vi "GetFunctionOptions.vi"(9 "Function in":refnum<class "Function.lvclass">) -> (3 "Function out":refnum<class "Function.lvclass">, 4 "options":string)   [LabVIEW 2014, in "Raspberry Pi Compatible Compiler for LabVIEW.lvlib" / "Function.lvclass"]
uses:
  Function.lvclass
  Python/Parsing/Python Functions.lvlib
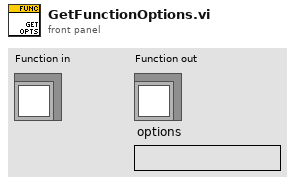
[diagram p1: front panel]
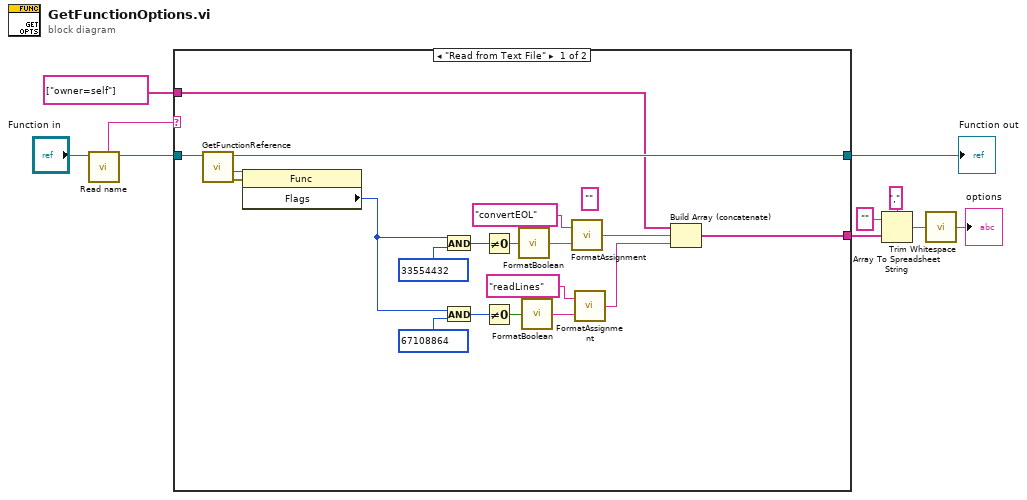
[diagram p0: block diagram]
diagram:
  n1 = call-dynamic "Read name.vi"("Node in"="Function in") -> ("Node out"=w4:refnum<class "Function.lvclass">, "name"=w9:string)  [unwired: 7 in]
  n2 = case shown="\"Read from Text File\"" w9 {
    tunnel: [w13 w30] -> w8
    tunnel: w4 -> [w29 w31]
    tunnel: [w12 w31] -> w3
    tunnel: string[] ["owner=self"] -> [w11 w30]
    frame "Read from Text File" {
      (unwired) "" ("element")
      n3 = call "GetFunctionReference.vi"("Function in"=w29) -> ("error out"=w27:errorcluster, "reference out"=w28:refnum<vi>, "Function out"=w12:refnum<class "Function.lvclass">)  [unwired: 8 in]
      n4 = property class="Func"(reference=w28, error in=w27) -> ("Flags"=w22:u32)  [unwired: 2 out]
      n5 = And(x=w22, y=u32 33554432) -> (x .and. y?=w25:u32)
      n6 = And(x=w22, y=u32 67108864) -> (x .and. y?=w24:u32)
      n7 = Not Equal To 0?(x=w25) -> (x != 0?=w16:bool)
      n8 = Not Equal To 0?(x=w24) -> (x != 0?=w17:bool)
      n9 = call "FormatBoolean.vi"("value"=w16) -> ("python object"=w21:string)
      n10 = call "FormatBoolean.vi"("value"=w17) -> ("python object"=w18:string)
      n11 = call "FormatAssignment.vi"("value"=w21, "name"="convertEOL") -> ("python assignment"=w15:string)
      n12 = call "FormatAssignment.vi"("value"=w18, "name"="readLines") -> ("python assignment"=w14:string)
      n13 = Build Array (concatenate)(w11, w15, w14) -> (w13:string[])
    }
    frame Default {
    }
  }
  "Function out" <- w3
  n14 = Array To Spreadsheet String(delimiter (Tab)=",", array=w8, 3:"" ("format string")) -> (spreadsheet string=w6:string)
  n15 = call <vilib>:"Trim Whitespace.vi"("string"=w6) -> ("trimmed string"=→"options":string)  [unwired: 1 in]
